vi "Query PRACH Modulation Extreme Limit Check Results.vi"(8 "error in (no error)":errorcluster, 10 "Instance (1)":T1=1, 11 "VISA resource name":refnum<visa-resource-name>) -> (0 "error out":errorcluster, 1 "Out Of Tolerance":i32, 2 "Reliability":i32, 3 "VISA resource name out":refnum<visa-resource-name>, 4 "Limit Check Results":i32[](array[numeric]))   [LabVIEW 2020, in "Rohde&Schwarz CMWXP NR FR1 Measurement.lvlib"]
doc: "Returns the limit check results for modulation extreme values.\n\nAttribute:\nRSCMWXPNRFR1M_ATTR_QUERY_PRACH_MODULATION_EXTREME_LIMIT_CHECK_RESULTS\n\nRemote-control command:\nCALCulate:NRSub:MEAS<i>:PRACh:MODulation:EXTReme?"
uses:
  <instrlib>/Rohde&Schwarz CMWXP NR FR1 Measurement/Rohde&Schwarz CMWXP NR FR1 Measurement.lvlib
  <instrlib>/Rohde&Schwarz CMWXP NR FR1 Measurement/Private/_Instance.ctl
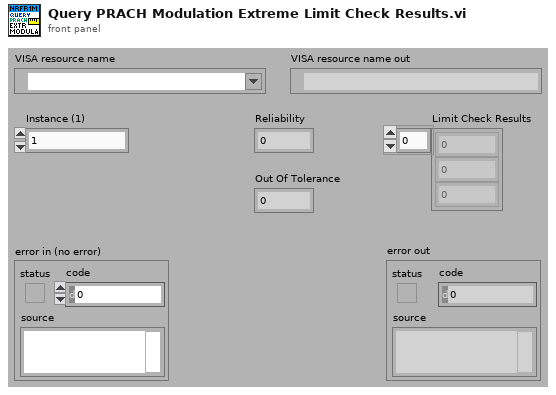
[diagram p1: front panel]
types:
  T1 = typedef "Rohde&Schwarz CMWXP NR FR1 Measurement.lvlib/_Instance.ctl" = i32
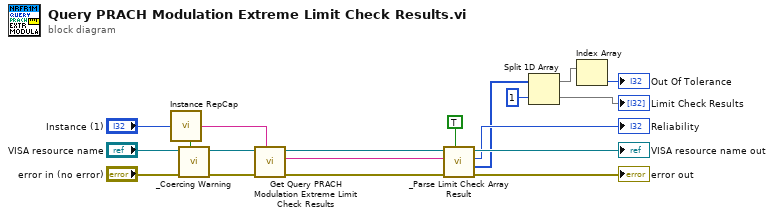
[diagram p0: block diagram]
diagram:
  n1 = call <instrlib>:"Instance RepCap.vi"("Instance In"="Instance (1)") -> ("In Range?"=w19:bool, "RepCap Identifier Out"=w13:string)  [unwired: 1 in]
  n2 = call <instrlib>:"_Coercing Warning.vi"("In Range?"=w19, "error in (no error)"="error in (no error)", "VISA resource name"="VISA resource name") -> ("error out"=w15:errorcluster, "VISA resource name out"=w14:refnum<visa-resource-name>)  [unwired: 7 in]
  n3 = call "Get Query PRACH Modulation Extreme Limit Check Results"("Repeated Capabilities"=w13, "error in (no error)"=w15, "instrument handle"=w14) -> ("error out"=w12:errorcluster, "Query PRACH Modulation Extreme Limit Check Results"=w8:string, "instrument handle out"=w9:refnum<visa-resource-name>)  [unwired: 6 in]
  n4 = call <instrlib>:"_Parse Limit Check Array Result.vi"("error in (no error)"=w12, "Input String"=w8, "VISA resource name"=w9, "Out of tolerance? (F)"=TRUE) -> ("error out"=→"error out":errorcluster, "Results"=w3:i32[], "Reliability"=→"Reliability":i32, "VISA resource name out"=→"VISA resource name out":refnum<visa-resource-name>)  [unwired: 2 in, 1 out]
  n5 = Split 1D Array(array=w3, index=1) -> (first subarray=w4:i32[], second subarray=→"Limit Check Results":i32[])
  n6 = Index Array(array=w4) -> (element=→"Out Of Tolerance":i32)  [unwired: 1 in]
